vi "Initialize Attributes.vi"(8 "error in (no error)":errorcluster, 10 "Attribute Data":variant, 11 "PVClient-Example in":refnum<class "PVClient-Example.lvclass">) -> (0 "error out":errorcluster, 2 "Found?":bool, 3 "PVClient-Example out":refnum<class "PVClient-Example.lvclass">)   [LabVIEW 2012, in "PVClient-Example.lvlib" / "PVClient-Example.lvclass"]
doc: "Initialize object attribute.\n\nUnique resources should be allocated elsewhere!"
uses:
  PVClient-Example.lvclass
  Core/Actors/CS++BaseActor/CS++BaseActor.lvclass
  PVClient-Example.lvclass/PVClient-Example.ctl
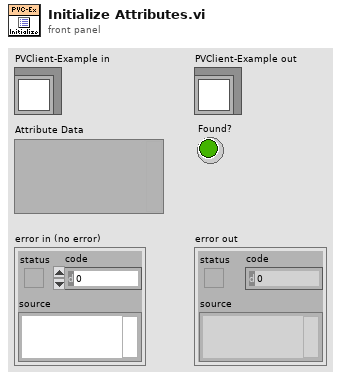
[diagram p1: front panel]
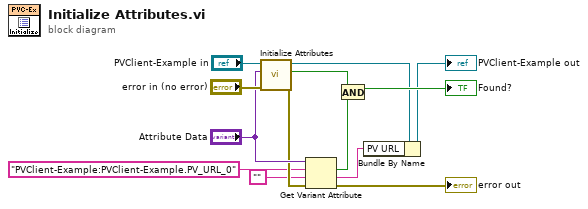
[diagram p0: block diagram]
diagram:
  n1 = call-parent "Initialize Attributes.vi"("error in (no error)"="error in (no error)", "Attribute Data"="Attribute Data", "CS++BaseActor in"="PVClient-Example in") -> ("error out"=w9:errorcluster, "Found?"=w13:bool, "CS++BaseActor out"=w2:refnum<class "PVClient-Example.lvclass">)  [unwired: 6 in]
  n2 = Get Variant Attribute(Variant="Attribute Data", name="PVClient-Example:PVClient-Example.PV_URL_0", default value (empty Variant)="", error in=w9) -> (found=w4:bool, value=w3:string, error out=→"error out":errorcluster)  [unwired: 1 out]
  n3 = And(x=w13, y=w4) -> (x .and. y?=→"Found?":bool)
  n4 = Bundle By Name(cluster=w2, "PV URL"=w3) -> (→"PVClient-Example out":refnum<class "PVClient-Example.lvclass">)
